vi "Actor Core.vi"(8 "error in":errorcluster, 11 "Splitter Settings UI in":refnum<class "Splitter Settings UI.lvclass">) -> (0 "error out":errorcluster, 3 "Actor out":refnum<class "Actor.lvclass">)   [LabVIEW 2015, in "Splitter Settings UI.lvlib" / "Splitter Settings UI.lvclass"]
doc: "The user interface for this panel.\n\n----\nPlease see the following web address for additional documentation and tutorial information:\nhttp://www.mooregoodideas.com/mgi-panel-manager/\n\nAuthor: Derek Trepanier\n\nCopyright (c) 2018, Moore Good Ideas, Inc.\n\nAll rights reserved.\n\nRedistribution and use in source and binary forms, with or without modification, are permitted provided that the following conditions are met:\n\n * Redistributions of source code must retain the above copyright notice, this list of conditions and the following disclaimer.\n * Redistributions in binary form must reproduce the above copyright notice, this list of conditions and the following disclaimer in the documentation and/or other materials provided with the distribution.\n * Neither the name of Moore Good Ideas, Inc. nor the names of its contributors may be used to endorse or promote products derived from this software without specific prior written permission.\n\nTHIS SOFTWARE IS PROVIDED BY THE COPYRIGHT HOLDERS AND CONTRIBUTORS \"AS IS\" AND ANY EXPRESS OR IMPLIED WARRANTIES, INCLUDING, BUT NOT LIMITED TO, THE IMPLIED WARRANTIES OF MERCHANTABILITY AND FITNESS FOR A PARTICULAR PURPOSE ARE DISCLAIMED. IN NO EVENT SHALL THE COPYRIGHT OWNER OR CONTRIBUTORS BE LIABLE FOR ANY DIRECT, INDIRECT, INCIDENTAL, SPECIAL, EXEMPLARY, OR CONSEQUENTIAL DAMAGES (INCLUDING, BUT NOT LIMITED TO, PROCUREMENT OF SUBSTITUTE GOODS OR SERVICES; LOSS OF USE, DATA, OR PROFITS; OR BUSINESS INTERRUPTION) HOWEVER CAUSED AND ON ANY THEORY OF LIABILITY, WHETHER IN CONTRACT, STRICT LIABILITY, OR TORT (INCLUDING NEGLIGENCE OR OTHERWISE) ARISING IN ANY WAY OUT OF THE USE OF THIS SOFTWARE, EVEN IF ADVISED OF THE POSSIBILITY OF SUCH DAMAGE."
uses:
  Splitter Settings UI.lvclass
  <vilib>/ActorFramework/Actor/Actor.lvclass
  Typedefs/Splitter Style--Enum.ctl
  Classes/Splitter/Splitter.lvclass
  <vilib>/ActorFramework/Actor/Actor.lvclass/Actor.ctl
  <vilib>/ActorFramework/Message Enqueuer/Message Enqueuer.lvclass/Message Enqueuer.ctl
  Splitter Settings UI.lvclass/Splitter Settings UI.ctl
  Splitter Settings UI Messages/Set Cursor Busy State Msg/Set Cursor Busy State Msg.lvclass/Set Cursor Busy State Msg.ctl
  <vilib>/ActorFramework/Message Enqueuer/Init from Existing Queue.vi
  <vilib>/ActorFramework/Message Enqueuer/Enqueue.vi
  <vilib>/ActorFramework/Message Priority Queue/Priority Enqueue.vi
  <vilib>/ActorFramework/Message Enqueuer/Message Enqueuer.lvclass
  Pane Relief Main UI/Pane Relief Main UI Messages/Panel Object Settings Changed Msg/Panel Object Settings Changed Msg.lvclass
  Splitter Settings UI Messages/Set Cursor Busy State Msg/Set Cursor Busy State Msg.lvclass
  <vilib>/MGI/Panel Manager/Panel Actor/Panel Actor/Panel Actor.lvclass
panel:
  in  "Label":string
  in  "Style":T1 items=["Modern", "Classic", "System", "NXG"]
  in  "Size":i32 min=0
  in  "Color":u32(colorbox)
  in  "Locked":bool
  in  "Sticks":u16(ring) items=["Top", "Bottom", "Proportions"]
  in  "Position":i32
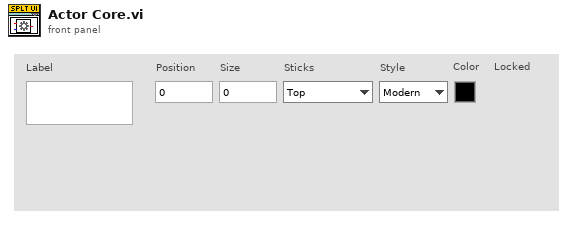
[diagram p1: front panel]
types:
  T1 = typedef "Splitter Style--Enum.ctl" = u16
  T2 = cluster{"Event Registration Refnum":refnum<event-registration>, "Pnl Actor":refnum<event-registration>}
  T3 = typedef "Splitter Sizing--Enum.ctl" = enum16{"Sticks Top/Left", "Sticks Bottom/Right", "Proportional"}
  T4 = typedef "Splitter Orientation--Enum.ctl" = enum16{"Vertical", "Horizontal"}
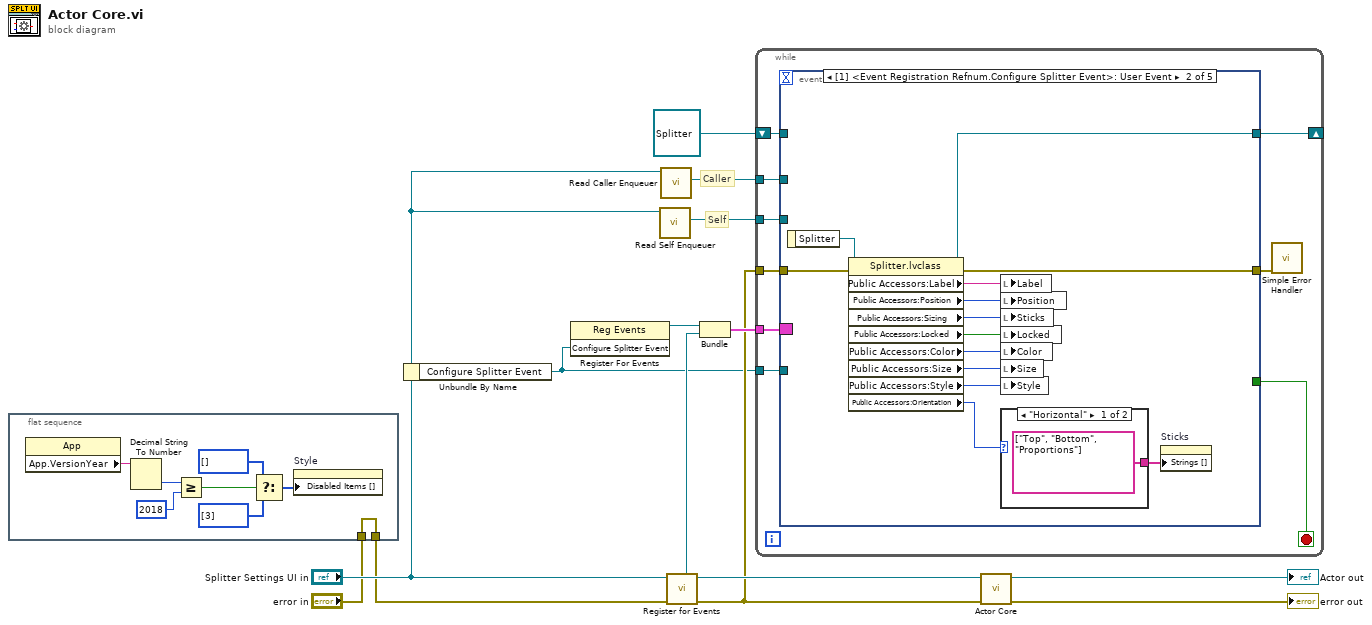
[diagram p0: block diagram]
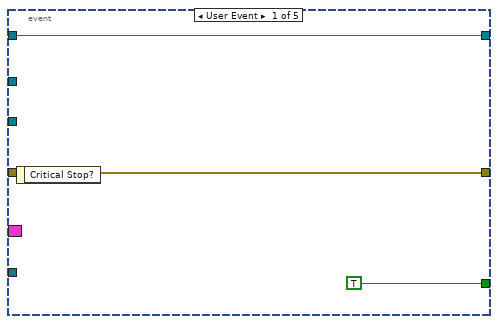
[diagram p2: hidden frame]
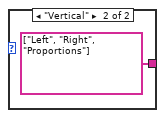
[diagram p3: hidden frame]
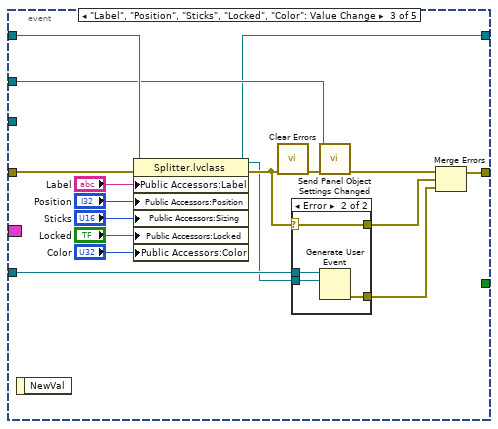
[diagram p4: hidden frame]
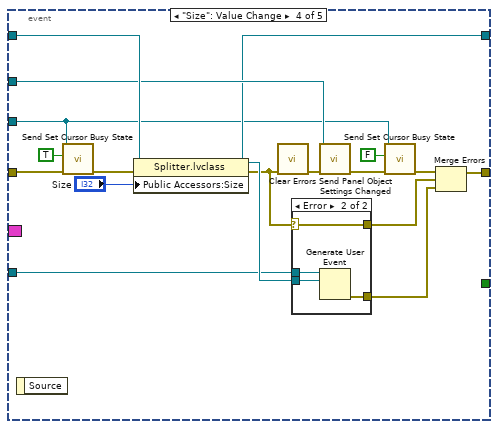
[diagram p6: hidden frame]
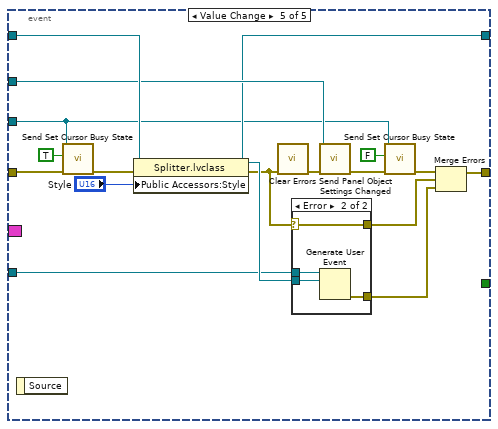
[diagram p8: hidden frame]
diagram:
  # "Self"
  # "Caller"
  n1 = flat-sequence {
    tunnel: [w15] -> w1
    tunnel: "error in" -> [w15]
    frame #0 {
      n2 = property class="App"() -> ("App.VersionYear"=w20:string)  [unwired: 2 in, 2 out]
      n3 = Decimal String To Number(string=w20) -> (number=w19:i32)  [unwired: 2 in, 1 out]
      n4 = Greater Or Equal?(x=w19, y=2018) -> (x >= y?=w17:bool)
      n5 = Select(t=i32[] [] ("Disabled Items []"), s=w17, f=i32[] [3] ("Disabled Items []")) -> (s? t:f=w16:i32[])
      n6 = property on="Style" class="Ring (strict)"("Disabled Items []"=w16) -> ()  [unwired: 2 in, 2 out]
    }
  }
  n7 = Unbundle By Name("Splitter Settings UI in") -> ("Configure Splitter Event"=w5:refnum<user-event>)
  n8 = register-events(w5) -> (reference out=w11:refnum<event-registration>)  [unwired: 2 in, 1 out]
  n9 = call <vilib>:"Read Self Enqueuer.vi"("Actor"="Splitter Settings UI in") -> ("Self Enqueuer"=w4:refnum<class "Message Enqueuer.lvclass">)  [unwired: 10 in]
  n10 = call <vilib>:"Read Caller Enqueuer.vi"("Actor"="Splitter Settings UI in") -> ("Caller Enqueuer"=w6:refnum<class "Message Enqueuer.lvclass">)  [unwired: 10 in]
  n11 = call <vilib>:"Register for Events.vi"("Error In"=w1, "Panel Actor in"="Splitter Settings UI in") -> ("Error Out"=w7:errorcluster, "Panel Actor out"=w12:refnum<class "Splitter Settings UI.lvclass">, "Pnl Actor"=w10:refnum<event-registration>)  [unwired: 6 in, 1 out]
  n12 = Bundle("Event Registration Refnum"=w11, "Pnl Actor"=w10) -> (w9:T2)  [unwired: 1 in]
  n13 = while {
    tunnel: w9 -> [w31]
    shift-right: [w29] -> _
    shift-left: refnum<class "Splitter.lvclass"> refnum ("Splitter.lvclass") -> [w28]
    tunnel: w6 -> [w26]
    tunnel: w7 -> [w27]
    tunnel: w5 -> [w24]
    tunnel: w4 -> [w23]
    stop <- w30 stop-if-true
    n14 = event shown="[1] <Event Registration Refnum.Configure Splitter Event>: User Event" {
      selector: w31 -> [_ _ _ _ _]
      dyn-events: _ -> [_ _ _ _ _]
      timeout: _ -> [_ _ _ _ _]
      tunnel: [TRUE _ _ _ _] -> w30
      tunnel: [w34 w35 w51 w80 w103] -> w29
      tunnel: w28 -> [w34 _ w59 w87 w109]
      tunnel: w27 -> [w33 w42 w60 w75 w98]
      tunnel: [w33 w41 w55 w84 w107] -> w25
      tunnel: w26 -> [_ _ w57 w83 w106]
      tunnel: w24 -> [_ _ w52 w78 w101]
      tunnel: w23 -> [_ _ _ w73 w96]
      event User Event {
        n15 = event-data() -> ()  [unwired: 1 in, 1 out]
      }
      event User Event {
        n16 = event-data() -> ("Splitter"=w36:refnum<class "Splitter.lvclass">)  [unwired: 1 in]
        n17 = property class="Splitter.lvclass"(reference=w36, error in=w42) -> (reference out=w35:refnum<class "Splitter.lvclass">, error out=w41:errorcluster, "Public Accessors:Label"=w47:string, "Public Accessors:Position"=w46:i32, "Public Accessors:Sizing"=w45:T3, "Public Accessors:Locked"=w44:bool, "Public Accessors:Color"=w43:u32, "Public Accessors:Size"=w40:i32, "Public Accessors:Style"=w37:T1, "Public Accessors:Orientation"=w38:T4)
        n18 = local write "Label"(w47) -> ()
        n19 = local write "Position"(w46) -> ()
        n20 = local write "Sticks"(w45) -> ()
        n21 = local write "Locked"(w44) -> ()
        n22 = local write "Color"(w43) -> ()
        n23 = local write "Size"(w40) -> ()
        n24 = local write "Style"(w37) -> ()
        n25 = case shown="\"Horizontal\"" w38 {
          tunnel: [string[] ["Top", "Bottom", "Proportions"] ("Strings []") string[] ["Left", "Right", "Proportions"] ("Strings []")] -> w39
          frame "Horizontal" {
          }
          frame "Vertical" {
          }
        }
        n26 = property on="Sticks" class="Ring (strict)"("Strings []"=w39) -> ()  [unwired: 2 in, 2 out]
      }
      event "Label", "Position", "Sticks", "Locked", "Color": Value Change {
        n27 = event-data() -> ()  [unwired: 1 in, 1 out]
        n28 = property class="Splitter.lvclass"(reference=w59, error in=w60, "Public Accessors:Label"="Label", "Public Accessors:Position"="Position", "Public Accessors:Sizing"="Sticks", "Public Accessors:Locked"="Locked", "Public Accessors:Color"="Color") -> (reference out=w51:refnum<class "Splitter.lvclass">, error out=w53:errorcluster)
        n29 = call <vilib>:"Clear Errors.vi"("error in (no error)"=w53) -> ("error out"=w58:errorcluster)  [unwired: 5 in, 1 out]
        n30 = case shown="Error" w53 {
          selector: w53 -> [w66 w70]
          tunnel: [w66 w70] -> w54
          tunnel: w52 -> [_ w69]
          tunnel: w51 -> [_ w68]
          tunnel: [_ w67] -> w50
          frame No Error {
          }
          frame Error {
            n31 = Generate User Event(user event=w69, event data cluster=w68) -> (error out=w67:errorcluster)  [unwired: 2 in, 1 out]
          }
        }
        n32 = call "Send Panel Object Settings Changed.vi"("error in (no error)"=w58, "Message Enqueuer"=w57) -> ("error out"=w56:errorcluster)  [unwired: 8 in, 1 out]
        n33 = Merge Errors(w56, w54, w50) -> (w55:errorcluster)
      }
      event "Size": Value Change {
        n34 = event-data() -> ()  [unwired: 1 in, 1 out]
        n35 = call "Send Set Cursor Busy State.vi"("error in (no error)"=w75, "Busy?"=TRUE, "Message Enqueuer"=w73) -> ("error out"=w76:errorcluster)  [unwired: 7 in, 1 out]
        n36 = property class="Splitter.lvclass"(reference=w87, error in=w76, "Public Accessors:Size"="Size") -> (reference out=w80:refnum<class "Splitter.lvclass">, error out=w79:errorcluster)
        n37 = call <vilib>:"Clear Errors.vi"("error in (no error)"=w79) -> ("error out"=w85:errorcluster)  [unwired: 5 in, 1 out]
        n38 = case shown="Error" w79 {
          selector: w79 -> [w88 w92]
          tunnel: [w88 w92] -> w82
          tunnel: w78 -> [_ w91]
          tunnel: w80 -> [_ w90]
          tunnel: [_ w89] -> w81
          frame No Error {
          }
          frame Error {
            n39 = Generate User Event(user event=w91, event data cluster=w90) -> (error out=w89:errorcluster)  [unwired: 2 in, 1 out]
          }
        }
        n40 = call "Send Panel Object Settings Changed.vi"("error in (no error)"=w85, "Message Enqueuer"=w83) -> ("error out"=w72:errorcluster)  [unwired: 8 in, 1 out]
        n41 = call "Send Set Cursor Busy State.vi"("error in (no error)"=w72, "Busy?"=FALSE, "Message Enqueuer"=w73) -> ("error out"=w71:errorcluster)  [unwired: 7 in, 1 out]
        n42 = Merge Errors(w71, w82, w81) -> (w84:errorcluster)
      }
      event Value Change {
        n43 = event-data() -> ()  [unwired: 1 in, 1 out]
        n44 = call "Send Set Cursor Busy State.vi"("error in (no error)"=w98, "Busy?"=TRUE, "Message Enqueuer"=w96) -> ("error out"=w99:errorcluster)  [unwired: 7 in, 1 out]
        n45 = property class="Splitter.lvclass"(reference=w109, error in=w99, "Public Accessors:Style"="Style") -> (reference out=w103:refnum<class "Splitter.lvclass">, error out=w102:errorcluster)
        n46 = call <vilib>:"Clear Errors.vi"("error in (no error)"=w102) -> ("error out"=w108:errorcluster)  [unwired: 5 in, 1 out]
        n47 = case shown="Error" w102 {
          selector: w102 -> [w110 w114]
          tunnel: [w110 w114] -> w105
          tunnel: w101 -> [_ w113]
          tunnel: w103 -> [_ w112]
          tunnel: [_ w111] -> w104
          frame No Error {
          }
          frame Error {
            n48 = Generate User Event(user event=w113, event data cluster=w112) -> (error out=w111:errorcluster)  [unwired: 2 in, 1 out]
          }
        }
        n49 = call "Send Panel Object Settings Changed.vi"("error in (no error)"=w108, "Message Enqueuer"=w106) -> ("error out"=w95:errorcluster)  [unwired: 8 in, 1 out]
        n50 = call "Send Set Cursor Busy State.vi"("error in (no error)"=w95, "Busy?"=FALSE, "Message Enqueuer"=w96) -> ("error out"=w94:errorcluster)  [unwired: 7 in, 1 out]
        n51 = Merge Errors(w94, w105, w104) -> (w107:errorcluster)
      }
    }
    n52 = call <vilib>:"Simple Error Handler.vi"("error in (no error)"=w25) -> ()  [unwired: 4 in, 5 out]
  }
  n53 = call-parent "Actor Core.vi"("error in"=w7, "Panel Actor in"=w12) -> ("error out"=→"error out":errorcluster, "Actor out"=→"Actor out":refnum<class "Actor.lvclass">)  [unwired: 8 in]
